vi "Strings.vi"(1 "#2":dbl=220.0, 2 "#1":dbl=110.0) -> (0 "Combinada":string="As tensoes sao: 110,0 220,0 volts")   [LabVIEW 2018]
panel:
  out "Numero out":dbl=110.0
  out "offset past match":i32=15
  out "after substring":string=" 110,0 220,0 volts"
  out "match substring":string=":"
  out "before substring":string="As tensoes sao"
  in  "String":string="As tensoes sao: 110,0 220,0 volts"
  out "Num elementos":dbl=33.0
  in  "Fim":string=" volts"
  in  "Início":string="As tensoes sao: "
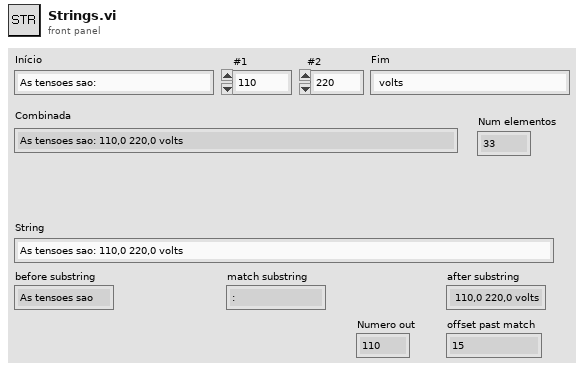
[diagram p1: front panel]
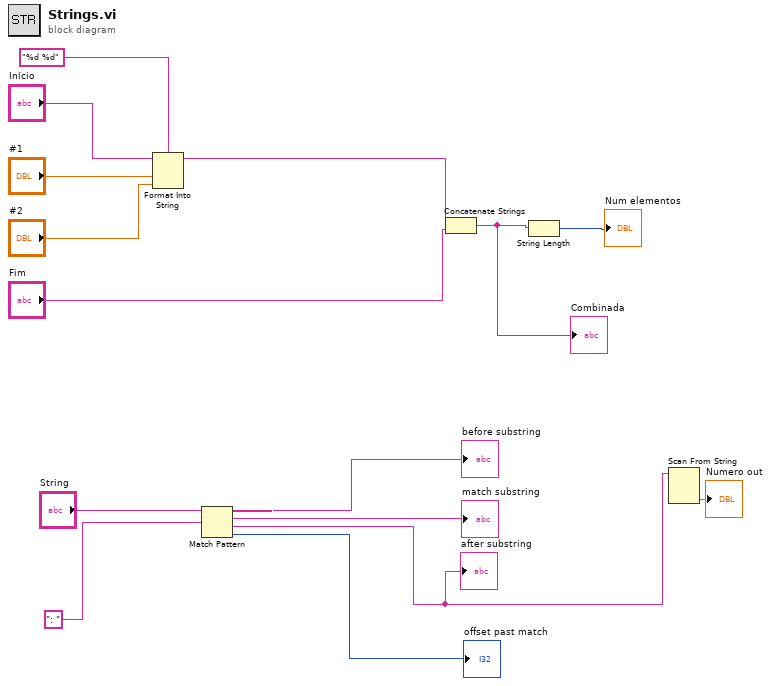
[diagram p0: block diagram]
diagram:
  n1 = Format Into String(format string="%d %d", initial string="Início", "#1", "#2") -> (resulting string=w13:string)  [unwired: 1 in, 1 out]
  n2 = Match Pattern(string="String", regular expression=": ") -> (before substring=→"before substring":string, match substring=→"match substring":string, after substring=w2:string, offset past match=→"offset past match":i32)  [unwired: 1 in]
  "after substring" <- w2
  n3 = Concatenate Strings(w13, "Fim") -> (w9:string)
  "Combinada" <- w9
  n4 = String Length(string=w9) -> (length=→"Num elementos":i32)
  n5 = Scan From String(input string=w2) -> (output 1=→"Numero out":dbl)  [unwired: 4 in, 3 out]
